vi "Output Arm.vi"(8 "error in (no error)":errorcluster, 11 "TeleOp Data Cluster":T1={"Drive Forward Input "=0.0, "Drive Twist Input"=0.0, "Drive Output"=0.0, "Drivetwist Output"=0.0, "Left Joystick Buttons"=[], "Left Joystick Axis"=[], "Right Joystick Axis"=[0.0, -0.007874015748031496, 0.0, 1.0], "Right Joystick Button"=[FALSE, FALSE, FALSE, FALSE, FALSE, FALSE, FALSE, FALSE, FALSE, FALSE, FALSE, FALSE], "Arm Encoder"=1.0, "Left Drive Encoder"=1.0, "Right Drive Encoder"=3.0, "Gyro Angle "=17.9296875, "Arm Joystick Output  "=-0.003937007874015748, "Line Follower L, C, R "=[TRUE, TRUE, TRUE], "Line follow?"=FALSE, " Climb Solenoid"=FALSE, "Wrist Encoder Count"=0.0, "Wrist Joystick Output"=0.0, "Ball Encoder Count"=0.0, "Ball Output"=0.0, "Climb Encoder"=0.0, "Climb Motor Output"=0.0, " Hatch Solenoid"=FALSE, "Arm Setpoint "=6.0, "Wrist Setpoint "=1.0, "Arm Joystick Enabled?"=FALSE, "Wrist Joystick Enabled"=FALSE, "Vision String"="0, 0, 0, 0, 0, 0", "Left Joystick POVs"=[]}) -> (0 "error out":errorcluster)   [LabVIEW 2018]
uses:
  TypeDefs/Teleop Data Cluster.ctl
  TypeDefs/typedef_enum_Refnums.ctl
  TypeDefs/Joystick Buttons.ctl
  <vilib>/Rock Robotics/WPI/ThirdParty/Phoenix-LabVIEW/Motor Controller/Controls/CTRE_Phoenix_MotorControl_ControlMode.ctl
  <vilib>/Rock Robotics/WPI/ThirdParty/Phoenix-LabVIEW/Motor Controller/Get/CTRE_Phoenix_MotorController_GetVoltage.vi
  <vilib>/Rock Robotics/WPI/ThirdParty/Phoenix-LabVIEW/Motor Controller/Get/CTRE_Phoenix_MotorController_GetClosedLoopData.vi
  <vilib>/Rock Robotics/WPI/ThirdParty/Phoenix-LabVIEW/Motor Controller/Get/CTRE_Phoenix_MotorController_GetQuadratureData.vi
  <vilib>/Rock Robotics/WPI/ThirdParty/Phoenix-LabVIEW/Motor Controller/Get/CTRE_Phoenix_MotorController_GetSelectedSensorData.vi
  <vilib>/Rock Robotics/Network Tables/NT Write Boolean.vi
  <vilib>/ptbypt/NI_PtbyPt.lvlib
panel:
  in  "Trigger":dbl=5.0
  in  "Setpoint 5":dbl=74.2
  in  "Setpoint 4":dbl=51.0
  in  "Setpoint 3":dbl=19.3
  in  "Setpoint 0":dbl=33.0
  in  "Setpoint 2":dbl=79.0
  in  "Setpoint 1":dbl=61.0
  in  "Position In":dbl=18.0 format="%#_13g"
  in  "Reset Encoder":bool
  out "velocity Chart":i32(graph)
  out "Encoder Count":dbl
  in  "Button Mode?":bool=TRUE
  out "Quadrature Velocity":i32
  in  "P":dbl=0.65
  in  "I":dbl
  in  "D":dbl=0.55
  in  "slotIdx":i32
  out "Encoder Graph":dbl[][](graph)=[[-19.990742000540358, 1.0]]
  out "Closed-loop Error":i32=-20
  out "Error Derivative":dbl
  out "Integral Accumulator":dbl=-59689.0
  out "Closed-loop Target":dbl=-0.019
  out "Percent Output":dbl
  in  "Cruise Angular Velocity raw":dbl=550.0 format="%#_13g"
  in  "Maximum Angular Accel raw":dbl=500.0 format="%#_13g"
  in  "F":dbl
  in  "Arbitrary Feed Forward at 0":dbl=0.23
  in  "joystick control? OR Thumb":bool
  # "ball"
  # "hatch"
  # "was 18.5"
  # "top:  button mode"
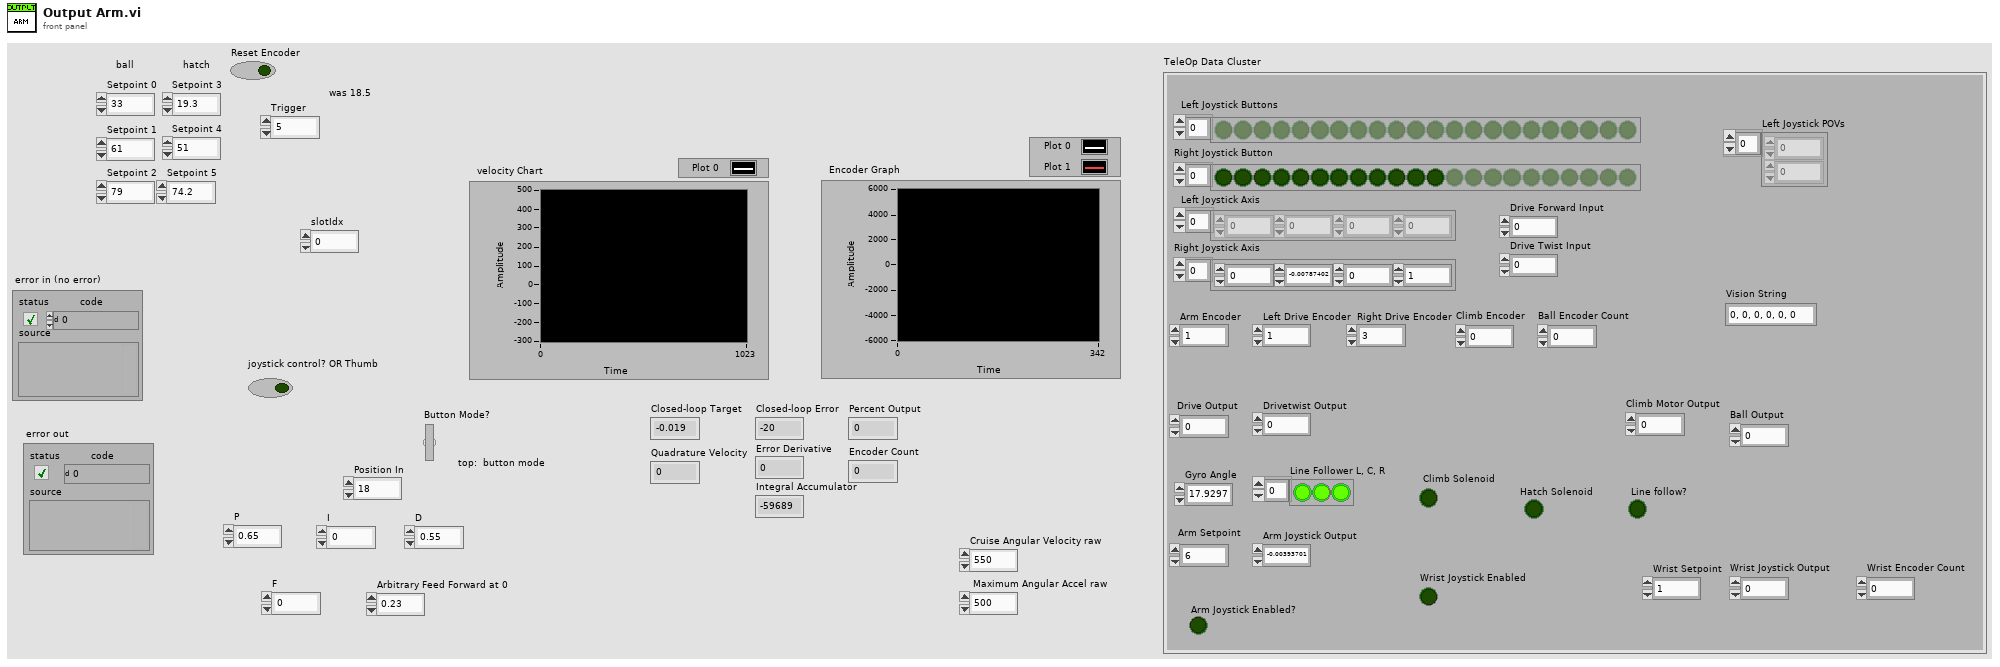
[diagram p1: front panel]
types:
  T1 = typedef "Teleop Data Cluster.ctl" = cluster{"Drive Forward Input ":dbl, "Drive Twist Input":dbl, "Drive Output":dbl, "Drivetwist Output":dbl, "Left Joystick Buttons":bool[], "Left Joystick Axis":dbl[], "Right Joystick Axis":dbl[], "Right Joystick Button":bool[], "Arm Encoder":dbl, "Left Drive Encoder":dbl, "Right Drive Encoder":dbl, "Gyro Angle ":dbl, "Arm Joystick Output  ":dbl, "Line Follower L, C, R ":bool[], "Line follow?":bool, " Climb Solenoid":bool, "Wrist Encoder Count":dbl, "Wrist Joystick Output":dbl, "Ball Encoder Count":dbl, "Ball Output":dbl, "Climb Encoder":dbl, "Climb Motor Output":dbl, " Hatch Solenoid":bool, "Arm Setpoint ":dbl, "Wrist Setpoint ":dbl, "Arm Joystick Enabled?":bool, "Wrist Joystick Enabled":bool, "Vision String":string, "Left Joystick POVs":i16[]}
  T2 = typedef "Joystick Buttons.ctl" = enum16{"Trigger", "Thumb", "Top 3", "Top 4", "Top 5", "Top 6", "Bottom 7", "Bottom 8", "Bottom 9", "Bottom 10", "Bottom 11", "Bottom 12"}
  T3 = typedef "typedef_enum_Refnums.ctl" = enum16{"Ball_Encoder", "Ball_Motor", "Camera", "Linefollow_3", "Linefollow_2", "Linefollow_1", "Gyro", "Hatch_Solenoid", "Climb_Back_Solenoid", "Arm_Encoder", "Arm_Motor", "Lift_Encoder", "Drive", "Drive_Motor_R", "Drive_Motor_L", "Drive_Encoder_R", "Drive_Encoder_L", "Joy_R", "Joy_L", "Wrist_Motor", "Wrist_Encoder", "Climb Upper Limit", "Climb Lower Limit ", "Climb_Front_Motor"}
  T4 = typedef "WPI_MotorControlDeviceRef.ctl" = cluster{"DeviceStatus":errorcluster, "Type":T5, "PWM":cluster{"PWM Channel":T6, "DeadBand":T7}, "CAN":cluster{"Device Number":u8, "SetOutput VI Ref":variant, "GetOutput VI Ref":variant, "Enable VI Ref":variant, "Disable VI Ref":variant, "Data":variant}, "Invert":bool, "DIO PWM":cluster{"PWM \"Enable\" Channel":T6, "DIOChannel":T8, "PWM Rate":dbl}}
  T5 = typedef "WPI_MotorControlType.ctl" = enum16{"PWM", "CAN", "DIO PWM"}
  T6 = typedef "FPGA_DIOPWMChannel.ctl" = enum8{"PWM 0", "PWM 1", "PWM 2", "PWM 3", "PWM 4", "PWM 5", "PWM 6", "PWM 7", "PWM 8", "PWM 9", "PWM MXP 0", "PWM MXP 1", "PWM MXP 2", "PWM MXP 3", "PWM MXP 4", "PWM MXP 5", "PWM MXP 6", "PWM MXP 7", "PWM MXP 8", "PWM MXP 9", "Invalid"}
  T7 = typedef "WPI_PWMDeadband.ctl" = cluster{"Name":string, "maxPositivePwm":i32, "minPositivePwm":i32, "centerPwm":i32, "maxNegativePwm":i32, "minNegativePwm":i32, "angularRange":u16}
  T8 = typedef "FPGA_DIOChannel.ctl" = enum8{"DIO 0", "DIO 1", "DIO 2", "DIO 3", "DIO 4", "DIO 5", "DIO 6", "DIO 7", "DIO 8", "DIO 9", "DIO MXP 0", "DIO MXP 1", "DIO MXP 2", "DIO MXP 3", "DIO MXP 4", "DIO MXP 5", "DIO MXP 6", "DIO MXP 7", "DIO MXP 8", "DIO MXP 9", "DIO MXP 10", "DIO MXP 11", "DIO MXP 12", "DIO MXP 13", "DIO MXP 14", "DIO MXP 15", "SPI Port CS1", "SPI Port CS2", "SPI Port CS3", "SPI Port MISO", "SPI Port MOSI", "Invalid"}
  T9 = enum16{"DemandType_Neutral", "DemandType_AuxPID", "DemandType_ArbitraryFeedForward"}
  T10 = typedef "CTRE_Phoenix_MotorControl_ControlMode.ctl" = u16
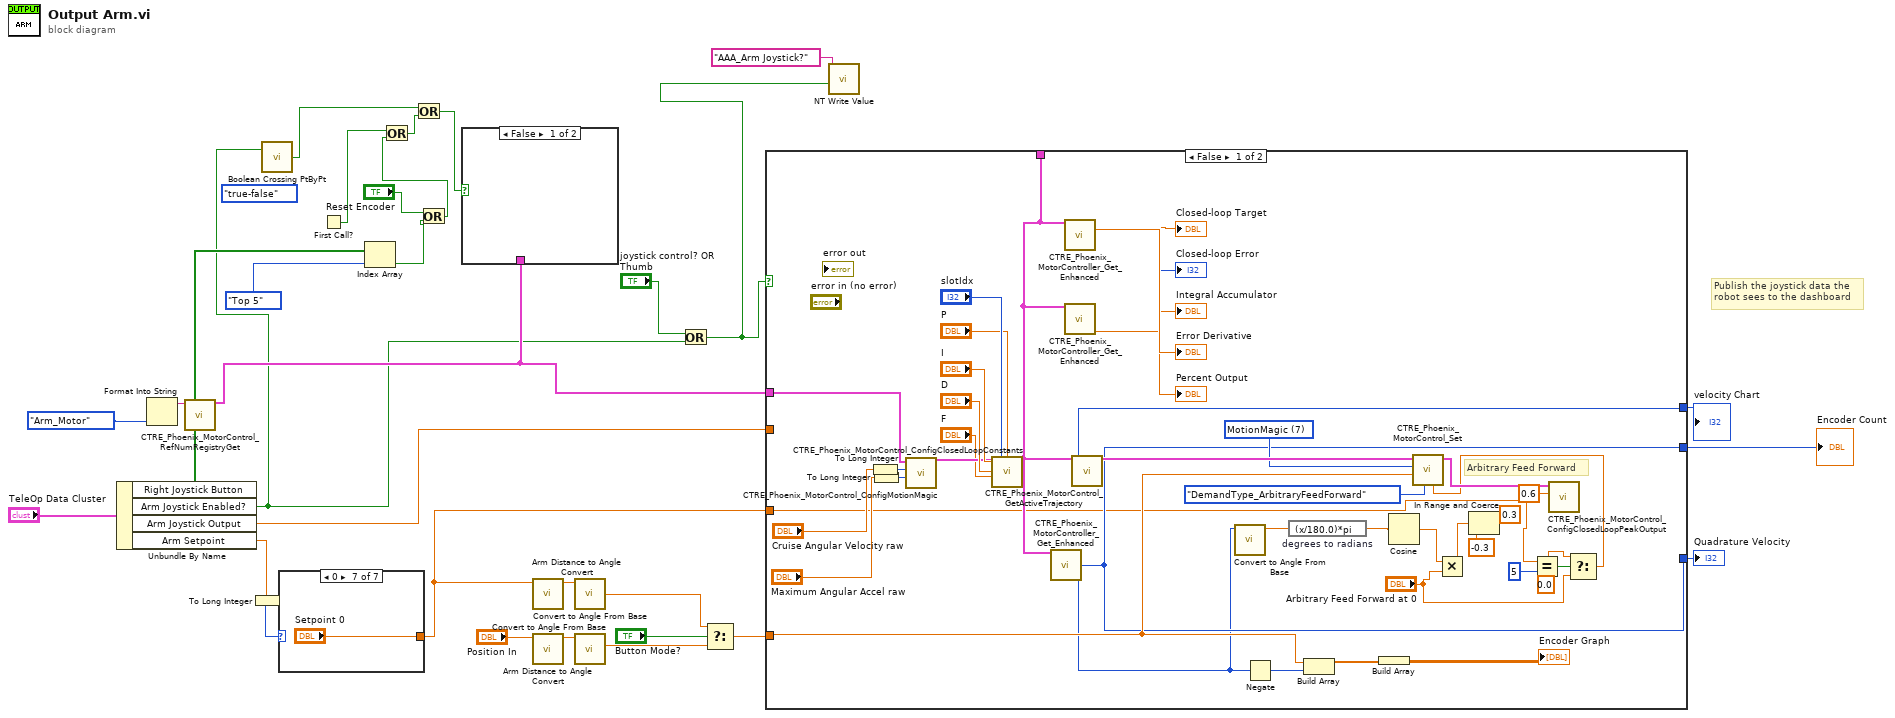
[diagram p0: block diagram]
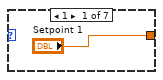
[diagram p2: hidden frame]
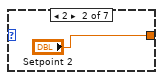
[diagram p3: hidden frame]
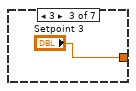
[diagram p4: hidden frame]
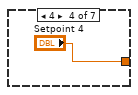
[diagram p5: hidden frame]
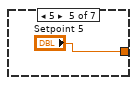
[diagram p6: hidden frame]
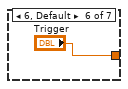
[diagram p7: hidden frame]
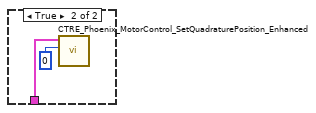
[diagram p8: hidden frame]
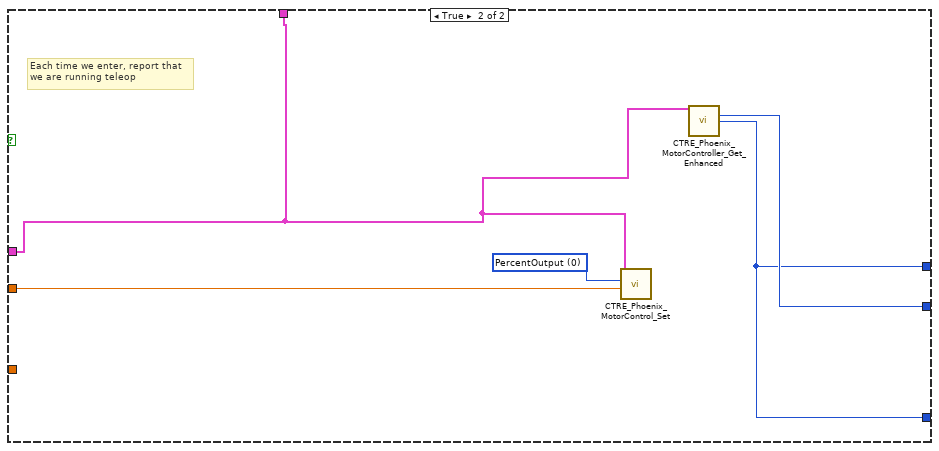
[diagram p9: hidden frame]
diagram:
  (unwired) enum16{"either", "false-true", "true-false"}."true-false" ("direction")
  # "Publish the joystick data the\nrobot sees to the dashboard"
  n1 = Unbundle By Name("TeleOp Data Cluster") -> ("Right Joystick Button"=w17:bool[], "Arm Joystick Enabled?"=w1:bool, "Arm Joystick Output"=w10:dbl, "Arm Setpoint"=w9:dbl)
  n2 = Format Into String(typedef_enum_Refnums."Arm_Motor" ("RefNums")) -> (resulting string=w26:string)  [unwired: 3 in, 1 out]
  n3 = call <vilib>:"CTRE_Phoenix_MotorControl_RefNumRegistryGet.vi"("refnum name"=w26) -> ("PhoenixMotorControlDevRef"=w5:T4)  [unwired: 9 in, 1 out]
  n4 = To Long Integer(number=w9) -> (32bit integer=w11:i32)
  n5 = call <vilib>:"Boolean Crossing PtByPt.vi"("input"=w1) -> ("crossing"=w3:bool)  [unwired: 2 in]
  n6 = case shown="0" w11 {
    tunnel: ["Setpoint 1" "Setpoint 2" "Setpoint 3" "Setpoint 4" "Setpoint 5" "Trigger" "Setpoint 0"] -> w8
    frame 1 {
    }
    frame 2 {
    }
    frame 3 {
    }
    frame 4 {
    }
    frame 5 {
    }
    frame 6, Default {
    }
    frame 0 {
    }
  }
  n7 = First Call?() -> (First Call?: T/F=w13:bool)
  n8 = Index Array(array=w17, index=Joystick_Buttons."Top 5" ("Enum")) -> (element=w16:bool)
  n9 = Or(x="Reset Encoder", y=w16) -> (x .or. y?=w12:bool)
  n10 = Or(x=w13, y=w12) -> (x .or. y?=w4:bool)
  n11 = Or(x=w3, y=w4) -> (x .or. y?=w2:bool)
  n12 = case shown="False" w2 {
    tunnel: w5 -> [_ w39]
    frame False {
    }
    frame True {
      n13 = call <vilib>:"CTRE_Phoenix_MotorControl_SetQuadraturePosition_Enhanced.vi"("New Position"=0, "PhoenixMotorControlDevRef"=w39) -> ()  [unwired: 8 in, 2 out]
    }
  }
  n14 = call "Arm Distance to Angle Convert.vi"("Distance In"=w8) -> ("Angle Out"=w21:dbl)  [unwired: 9 in, 1 out]
  n15 = call "Arm Distance to Angle Convert.vi"("Distance In"="Position In") -> ("Angle Out"=w22:dbl)  [unwired: 9 in, 1 out]
  n16 = call "Convert to Angle From Base.vi"("Angle In"=w21) -> ("Encoder Count Out"=w20:dbl)  [unwired: 9 in, 1 out]
  n17 = call "Convert to Angle From Base.vi"("Angle In"=w22) -> ("Encoder Count Out"=w25:dbl)  [unwired: 9 in, 1 out]
  n18 = Or(x="joystick control? OR Thumb", y=w1) -> (x .or. y?=w7:bool)
  n19 = Select(t=w20, s="Button Mode?", f=w25) -> (s? t:f=w28:dbl)
  n20 = case shown="False" w7 {
    tunnel: w28 -> [w74 _]
    tunnel: [w70 w84] -> w31
    tunnel: [w50 w84] -> w29
    tunnel: [w70 w85] -> w14
    tunnel: w10 -> [_ w83]
    tunnel: w5 -> [w51 w82]
    tunnel: [w49 w82] -> _
    tunnel: w8 -> [w46 _]
    frame False {
      w75 = T10 7 items=["PercentOutput"=0, "Position"=1, "Velocity"=2, "Current"=3, "Follower"=5, "MotionProfile"=6, "MotionMagic"=7, "MotionProfileArc"=10, "Disabled"=15] ("Control Mode")
      # "Arbitrary Feed Forward"
      n21 = To Long Integer(number="Cruise Angular Velocity raw") -> (32bit integer=w68:i32)
      n22 = To Long Integer(number="Maximum Angular Accel raw") -> (32bit integer=w67:i32)
      n23 = call <vilib>:"CTRE_Phoenix_MotorControl_ConfigMotionMagic.vi"("Acceleration"=w67, "Cruise Velocity"=w68, "PhoenixMotorControlDevRef"=w51) -> ("PhoenixMotorControlDevRef"=w76:T4)  [unwired: 7 in, 1 out]
      n24 = call <vilib>:"CTRE_Phoenix_MotorControl_ConfigClosedLoopConstants.vi"("PhoenixMotorControlDevRef"=w76, "slotIdx"="slotIdx", "P"="P", "I"="I", "D"="D", "F"="F") -> ("PhoenixMotorControlDevRef"=w49:T4)  [unwired: 8 in, 1 out]
      n25 = call-poly <vilib>:"CTRE_Phoenix_MotorController_Get_Enhanced.vi"("PhoenixMotorControlDevRef"=w49) -> ("Quadrature Position"=w56:i32, "Quadrature Velocity"=w70:i32)  [unwired: 11 in, 2 out]
      n26 = call-poly <vilib>:"CTRE_Phoenix_MotorController_Get_Enhanced.vi"("PhoenixMotorControlDevRef"=w49) -> ("Closed-loop Target"=→"Closed-loop Target":dbl, "Closed-loop Error"=→"Closed-loop Error":i32, "Error Derivative"=→"Error Derivative":dbl, "Integral Accumulator"=→"Integral Accumulator":dbl)  [unwired: 9 in, 2 out]
      n27 = call-poly <vilib>:"CTRE_Phoenix_MotorController_Get_Enhanced.vi"("PhoenixMotorControlDevRef"=w49) -> ("Percent Output"=→"Percent Output":dbl)  [unwired: 10 in, 4 out]
      n28 = call <vilib>:"CTRE_Phoenix_MotorControl_GetActiveTrajectory.vi"("PhoenixMotorControlDevRef"=w49) -> ("PhoenixMotorControlDevRef"=w80:T4, "Velocity (Sensor Units per 100 ms)"=w50:i32)  [unwired: 10 in, 3 out]
      n29 = call "Convert to Angle From Base.vi"("Horizontal Encoder Ct"=w56) -> ("Angle Out"=w57:dbl)  [unwired: 9 in, 1 out]
      n30 = Negate(x=w56) -> (-x=w52:i32)
      n31 = expression code="(x/180.0)*pi" "degrees to radians"(w57) -> (w58:dbl)
      n32 = Build Array(w74, w52) -> (w66:dbl[])
      n33 = Build Array(w66) -> (→"Encoder Graph":dbl[][])
      n34 = Cosine(x=w58) -> (cos(x)=w55:dbl)
      n35 = Multiply(x=w55, y="Arbitrary Feed Forward at 0") -> (x*y=w54:dbl)
      n36 = In Range and Coerce(upper limit=0.3, x=w54, lower limit=-0.3) -> ()  [unwired: 2 out]
      n37 = Equal?(x=w46, y=5) -> (x = y?=w44:bool)
      n38 = Select(t=0.0 ("f"), s=w44, f="Arbitrary Feed Forward at 0") -> (s? t:f=w43:dbl)
      n39 = call <vilib>:"CTRE_Phoenix_MotorControl_Set.vi"("Demand1"=w43, "DemandType"=T9."DemandType_ArbitraryFeedForward", "Output"=w74, "Control Mode"=w75, "PhoenixMotorControlDevRef"=w80) -> ("PhoenixMotorControlDevRef"=w61:T4)  [unwired: 5 in, 1 out]
      n40 = call <vilib>:"CTRE_Phoenix_MotorControl_ConfigClosedLoopPeakOutput.vi"("peakOutput"=0.6, "PhoenixMotorControlDevRef"=w61) -> ()  [unwired: 8 in, 2 out]
    }
    frame True {
      w86 = T10 0 items=["PercentOutput"=0, "Position"=1, "Velocity"=2, "Current"=3, "Follower"=5, "MotionProfile"=6, "MotionMagic"=7, "MotionProfileArc"=10, "Disabled"=15] ("Control Mode")
      # "Each time we enter, report that\nwe are running teleop"
      n41 = call <vilib>:"CTRE_Phoenix_MotorControl_Set.vi"("Output"=w83, "Control Mode"=w86, "PhoenixMotorControlDevRef"=w82) -> ()  [unwired: 7 in, 2 out]
      n42 = call-poly <vilib>:"CTRE_Phoenix_MotorController_Get_Enhanced.vi"("PhoenixMotorControlDevRef"=w82) -> ("Position (Raw Sensor Units)"=w85:i32, "Velocity (Raw Sensor Units per 100 ms)"=w84:i32)  [unwired: 11 in, 2 out]
    }
  }
  "Quadrature Velocity" <- w31
  "Encoder Count" <- w14
  "velocity Chart" <- w29
  n43 = call-poly <vilib>:"NT Write Value.vi"("Boolean"=w7, "Name"="AAA_Arm Joystick?") -> ()  [unwired: 9 in, 1 out]
